vi "INTELLIFAUCET AO Control.vi"(0 "VISA session":refnum<visa-resource-name>="MW100", 5 "HEWH MW100 Channel Numbers":T1="001", 7 "Output Value (0)":i32, 11 "Error In":errorcluster, 13 "milliseconds to wait":u32=100) -> (4 "dup VISA session":refnum<visa-resource-name>, 15 "error out":errorcluster)   [LabVIEW 2016]
uses:
  MW100/Type Definitions/HEWH MW100 Channel Numbers.ctl
panel:
  in  "Retries Allowed":i32=3
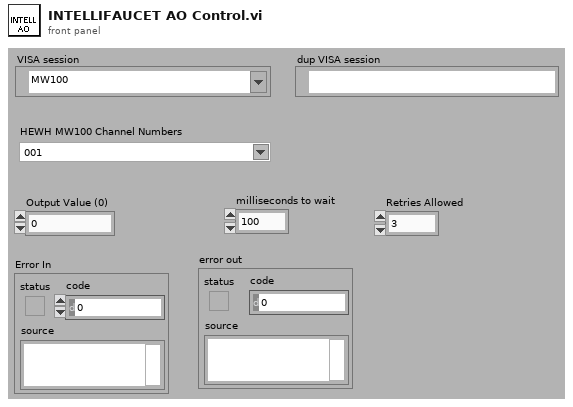
[diagram p1: front panel]
types:
  T1 = typedef "HEWH MW100 Channel Numbers.ctl" = string
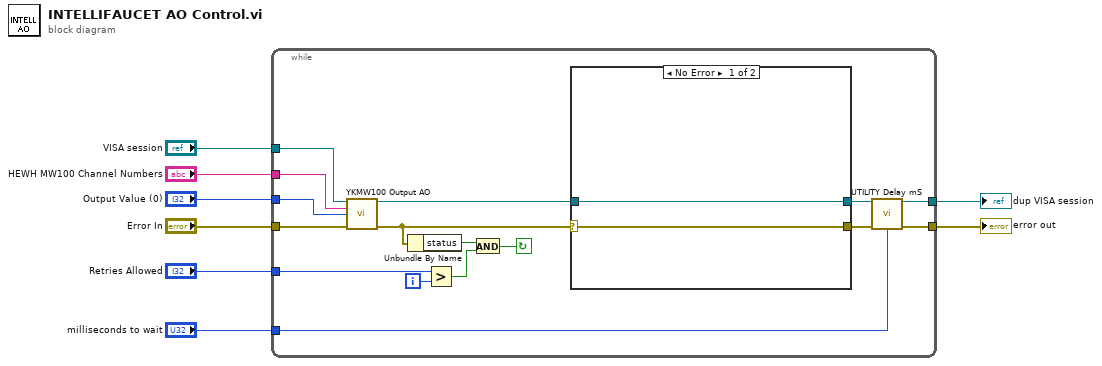
[diagram p0: block diagram]
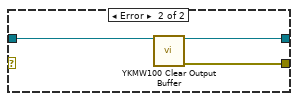
[diagram p2: hidden frame]
diagram:
  n1 = while {
    tunnel: "HEWH MW100 Channel Numbers" -> [w23]
    tunnel: "Output Value (0)" -> [w22]
    tunnel: "Error In" -> [w17]
    tunnel: [w10] -> w5
    tunnel: [w18] -> w8
    tunnel: "VISA session" -> [w21]
    tunnel: "Retries Allowed" -> [w13]
    tunnel: "milliseconds to wait" -> [w9]
    i -> [w15]
    stop <- w20 continue-if-true
    n2 = call "YKMW100 Output AO.vi"("VISA session"=w21, "Channel String (001)"=w23, "Output Value (0)"=w22, "error in (no error)"=w17) -> ("dup VISA session"=w11:refnum<visa-resource-name>, "error out"=w16:errorcluster)  [unwired: 10 in]
    n3 = Unbundle By Name(w16) -> ("status"=w19:bool)
    n4 = Greater?(x=w13, y=w15) -> (0:w14:bool)
    n5 = And(x=w19, y=w14) -> (x .and. y?=w20:bool)
    n6 = case shown="No Error" w16 {
      selector: w16 -> [w25 _]
      tunnel: w11 -> [w24 w28]
      tunnel: [w25 w26] -> w12
      tunnel: [w24 w27] -> w10
      frame No Error {
      }
      frame Error {
        n7 = call "YKMW100 Clear Output Buffer.vi"("VISA session"=w28) -> ("dup VISA session"=w27:refnum<visa-resource-name>, "error out"=w26:errorcluster)  [unwired: 13 in]
      }
    }
    n8 = call "UTILITY Delay mS.vi"("Error In"=w12, "milliseconds to wait"=w9) -> ("Error Out"=w18:errorcluster)  [unwired: 13 in]
  }
  "error out" <- w8
  "dup VISA session" <- w5
